vi "INIT SetFrameProperties.vi"(8 "error in (no error)":errorcluster, 11 "Device Item Ref in":T1 format="%.0x") -> (0 "error out":errorcluster, 3 "Device Item Ref out":T1 format="%.0x")   [LabVIEW 2018, in "CAN Gateway System Explorer.lvlib"]
uses:
  CAN Gateway System Explorer.lvlib
  <vilib>/NI Veristand/Custom Device API/Custom Device Item Ref.ctl
  Shared/Constants.vi
  <vilib>/NI Veristand/Custom Device API/Set Item Property (Variant).vi
  <vilib>/NI Veristand/Custom Device API/Custom Device API.lvlib
  Shared/CAN Gateway Shared.lvlib
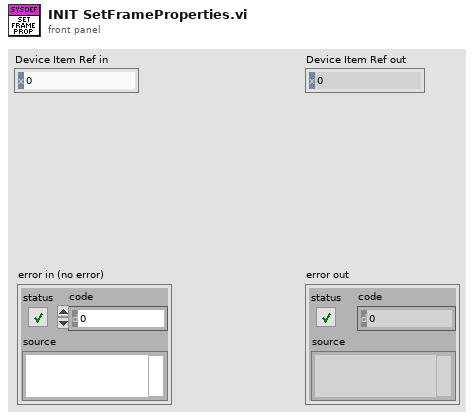
[diagram p1: front panel]
types:
  T1 = typedef "Custom Device API.lvlib/Custom Device Item Ref.ctl" = u64
  T2 = typedef "CAN Gateway System Explorer.lvlib/FramesCluster.ctl" = cluster{"Frame":string, "Fault":bool}
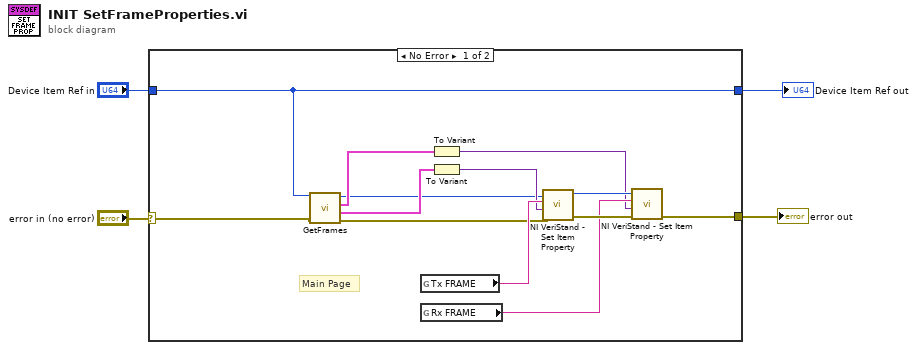
[diagram p0: block diagram]
diagram:
  n1 = case shown="No Error" "error in (no error)" {
    selector: "error in (no error)" -> [w12 w18]
    tunnel: "Device Item Ref in" -> [w7 w19]
    tunnel: [w14 w18] -> w2
    tunnel: [w7 w19] -> w1
    frame No Error {
      # "Main Page"
      n2 = call "GetFrames.vi"("error in (no error)"=w12, "Device Item Ref in"=w7) -> ("error out"=w5:errorcluster, "Tx Frames"=w10:T2[], "Rx Frames"=w11:T2[], "Device Item Ref out"=w6:T1)  [unwired: 6 in]
      n3 = global read "Constants.vi" "Tx FRAME"() -> (w17:string)
      n4 = global read "Constants.vi" "Rx FRAME"() -> (w15:string)
      n5 = To Variant(anything=w11) -> (Variant=w8:variant)
      n6 = To Variant(anything=w10) -> (Variant=w9:variant)
      n7 = call-poly <vilib>:"NI VeriStand - Set Item Property.vi"("error in (no error)"=w5, "Value"=w9, "Property Name"=w17, "Item Ref in"=w6) -> ("error out"=w16:errorcluster, "Item Ref out"=w13:T1)  [unwired: 5 in, 1 out]
      n8 = call-poly <vilib>:"NI VeriStand - Set Item Property.vi"("error in (no error)"=w16, "Value"=w8, "Property Name"=w15, "Item Ref in"=w13) -> ("error out"=w14:errorcluster)  [unwired: 5 in, 2 out]
    }
    frame Error {
    }
  }
  "error out" <- w2
  "Device Item Ref out" <- w1
